vi "initialize digest.vi"(8 "error in":errorcluster, 11 "digest name":string) -> (0 "error out":errorcluster, 3 "lvlibcrypto digest out":refnum<class "lvlibcrypto digest.lvclass">)   [LabVIEW 2016, in "lvlibcrypto digest.lvclass"]
uses:
  lvlibcrypto digest.lvclass
  lvlibcrypto digest.lvclass/lvlibcrypto digest.ctl
  lv tls dll.lvlib
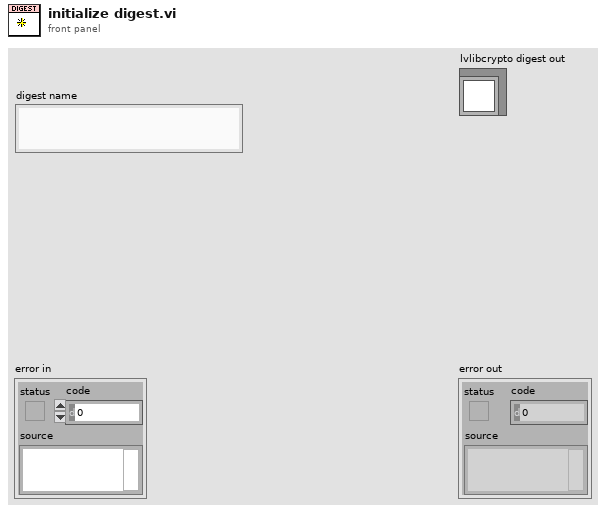
[diagram p1: front panel]
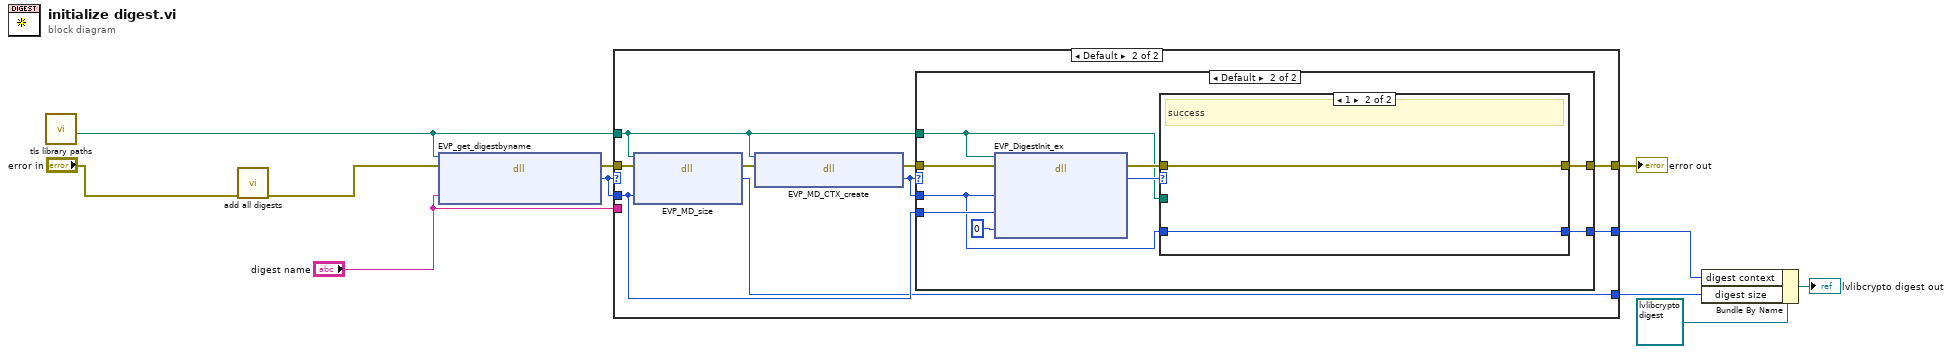
[diagram p0: block diagram]
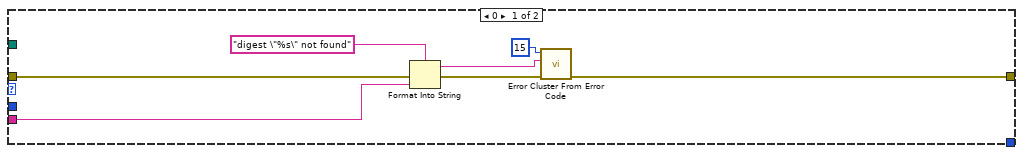
[diagram p2: hidden frame]
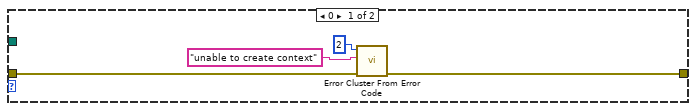
[diagram p3: hidden frame]
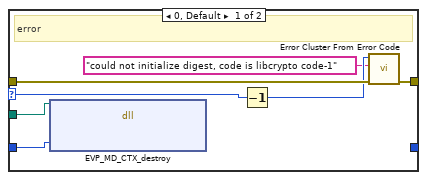
[diagram p4: hidden frame]
diagram:
  n1 = call "tls library paths.vi"() -> ("libcrypto"=w2:path)  [unwired: 8 in, 3 out]
  n2 = call "add all digests.vi"("error in"="error in") -> ("error out"=w3:errorcluster)  [unwired: 10 in]
  n3 = dll-call lib="C:/Users/IEUser/Desktop/tlssimple/libcrypto-41.dll" fn="EVP_get_digestbyname"(path in=w2, error in=w3, "digestname"="digest name") -> (error out=w10:errorcluster, "md"=w7:u64)  [unwired: 2 in, 1 out]
  n4 = case shown="Default" w7 {
    tunnel: w10 -> [w18 w23]
    tunnel: w2 -> [_ w21]
    tunnel: [w17 w26] -> w9
    tunnel: "digest name" -> [w13 _]
    tunnel: w7 -> [_ w20]
    tunnel: [_ w24] -> w5
    tunnel: [_ w19] -> w1
    frame 0 {
      n5 = Format Into String(format string="digest \"%s\" not found", error in=w18, w13) -> (resulting string=w14:string, error out=w15:errorcluster)  [unwired: 1 in]
      n6 = call <vilib>:"Error Cluster From Error Code.vi"("error in (no error)"=w15, "error message (\"\")"=w14, "error code (0)"=15) -> ("error out"=w17:errorcluster)  [unwired: 6 in]
    }
    frame Default {
      n7 = dll-call lib="C:/Users/IEUser/Desktop/tlssimple/libcrypto-41.dll" fn="EVP_MD_size"(path in=w21, error in=w23, "md"=w20) -> (error out=w22:errorcluster, "size"=w19:i32)  [unwired: 2 in, 1 out]
      n8 = dll-call lib="C:/Users/IEUser/Desktop/tlssimple/libcrypto-41.dll" fn="EVP_MD_CTX_create"(path in=w21, error in=w22) -> (error out=w27:errorcluster, "context"=w25:u64)  [unwired: 1 in, 1 out]
      n9 = case shown="Default" w25 {
        tunnel: w27 -> [w31 w40]
        tunnel: [w30 w36] -> w26
        tunnel: w25 -> [_ w33]
        tunnel: w20 -> [_ w38]
        tunnel: w21 -> [_ w34]
        tunnel: [_ w32] -> w24
        frame 0 {
          n10 = call <vilib>:"Error Cluster From Error Code.vi"("error in (no error)"=w31, "error message (\"\")"="unable to create context" ("error message (\"\")"), "error code (0)"=2) -> ("error out"=w30:errorcluster)  [unwired: 6 in]
        }
        frame Default {
          n11 = dll-call lib="C:/Users/IEUser/Desktop/tlssimple/libcrypto-41.dll" fn="EVP_DigestInit_ex"(path in=w34, error in=w40, "context"=w33, "digesttype"=w38, "engine null"=u64 0) -> (error out=w35:errorcluster, "ret"=w37:i32)  [unwired: 4 in, 1 out]
          n12 = case shown="1" w37 {
            selector: w37 -> [w45 _]
            tunnel: [w46 w49] -> w36
            tunnel: w35 -> [w47 w49]
            tunnel: w34 -> [w42 _]
            tunnel: w33 -> [w41 w48]
            tunnel: [_ w48] -> w32
            frame 0, Default {
              # "error"
              n13 = dll-call lib="C:/Users/IEUser/Desktop/tlssimple/libcrypto-41.dll" fn="EVP_MD_CTX_destroy"(path in=w42, "context"=w41) -> ()  [unwired: 4 in, 2 out]
              n14 = Decrement(x=w45) -> (x-1=w44:i32)
              n15 = call <vilib>:"Error Cluster From Error Code.vi"("error in (no error)"=w47, "error message (\"\")"="could not initialize digest, code is libcrypto code-1" ("error message (\"\")"), "error code (0)"=w44) -> ("error out"=w46:errorcluster)  [unwired: 6 in]
            }
            frame 1 {
              # "success"
            }
          }
        }
      }
    }
  }
  "error out" <- w9
  n16 = Bundle By Name(cluster=refnum<class "lvlibcrypto digest.lvclass"> refnum ("lvlibcrypto digest in"), "digest context"=w5, "digest size"=w1) -> (→"lvlibcrypto digest out":refnum<class "lvlibcrypto digest.lvclass">)
